vi "pulse_tester_16IQ.vi"() -> ()   [LabVIEW 2022 SP3]
uses:
  <vilib>/Analysis/NI_AALPro.lvlib
  <vilib>/measure/NI_MAPro.lvlib
  <vilib>/measure/maspectr.llb/FFT Power Spectrum and PSD for 1 Chan (CDB).vi
  <instrlib>/_niInstr/Basic Elements/v1/FPGA/niInstr Basic Elements v1 FPGA.lvlib
  emitter params.ctl
  pdw.ctl
  mode_type.ctl
panel:
  out "D phase to Dt":dbl[](graph)
  out "output valid":i16[](graph)
  in  "tx rate":i32=50
  out "Cluster":T1={"PW"=60000, "frequency shift"=0.004999999999999005, "amp"=0.31623077392578125, "mode type"=enum."LFM", "mode depth"=234562481, "mode filter"=0, "phase shift"=0.0}
  out "Array":i32[](array[numeric])
  out "free DDS":i16[](graph)
  out "Power Spectrum / PSD":cluster{"f0":dbl, "df":dbl, "magnitude":dbl[]}[](graph)
  out "amp out":dbl[](graph)
  out "phase out":dbl[](graph)
  in  "num of sampels for test":i32=65000 format="%.0p"
  out "I data":dbl[](graph)
  in  "emmiter":T3[](array[typedef])=[{"f set"=[1000000.0], "hop rate (Hz)"=6000.0, "d.c."=0.9, "amp (dB)"=-10.0, "mod type"=enum."LFM", "mod depth"=10000000.0, "DOA"=0.0, "t start"=0.0, "t end"=0.0}] {"t end" format="%#_3p"; "t start" format="%#_3p"; "DOA" format="%#_3p"; "mod depth" format="%.0p"}
  out "phase in to DDS":dbl[](graph)
  out "frequncy  in to DDS":dbl[](graph)
  in  "Fs":i32=200000000 format="%.0p"
  # "mode type:\n0- cw\n3-lfm\n4- bpsk\n5-qpsk"
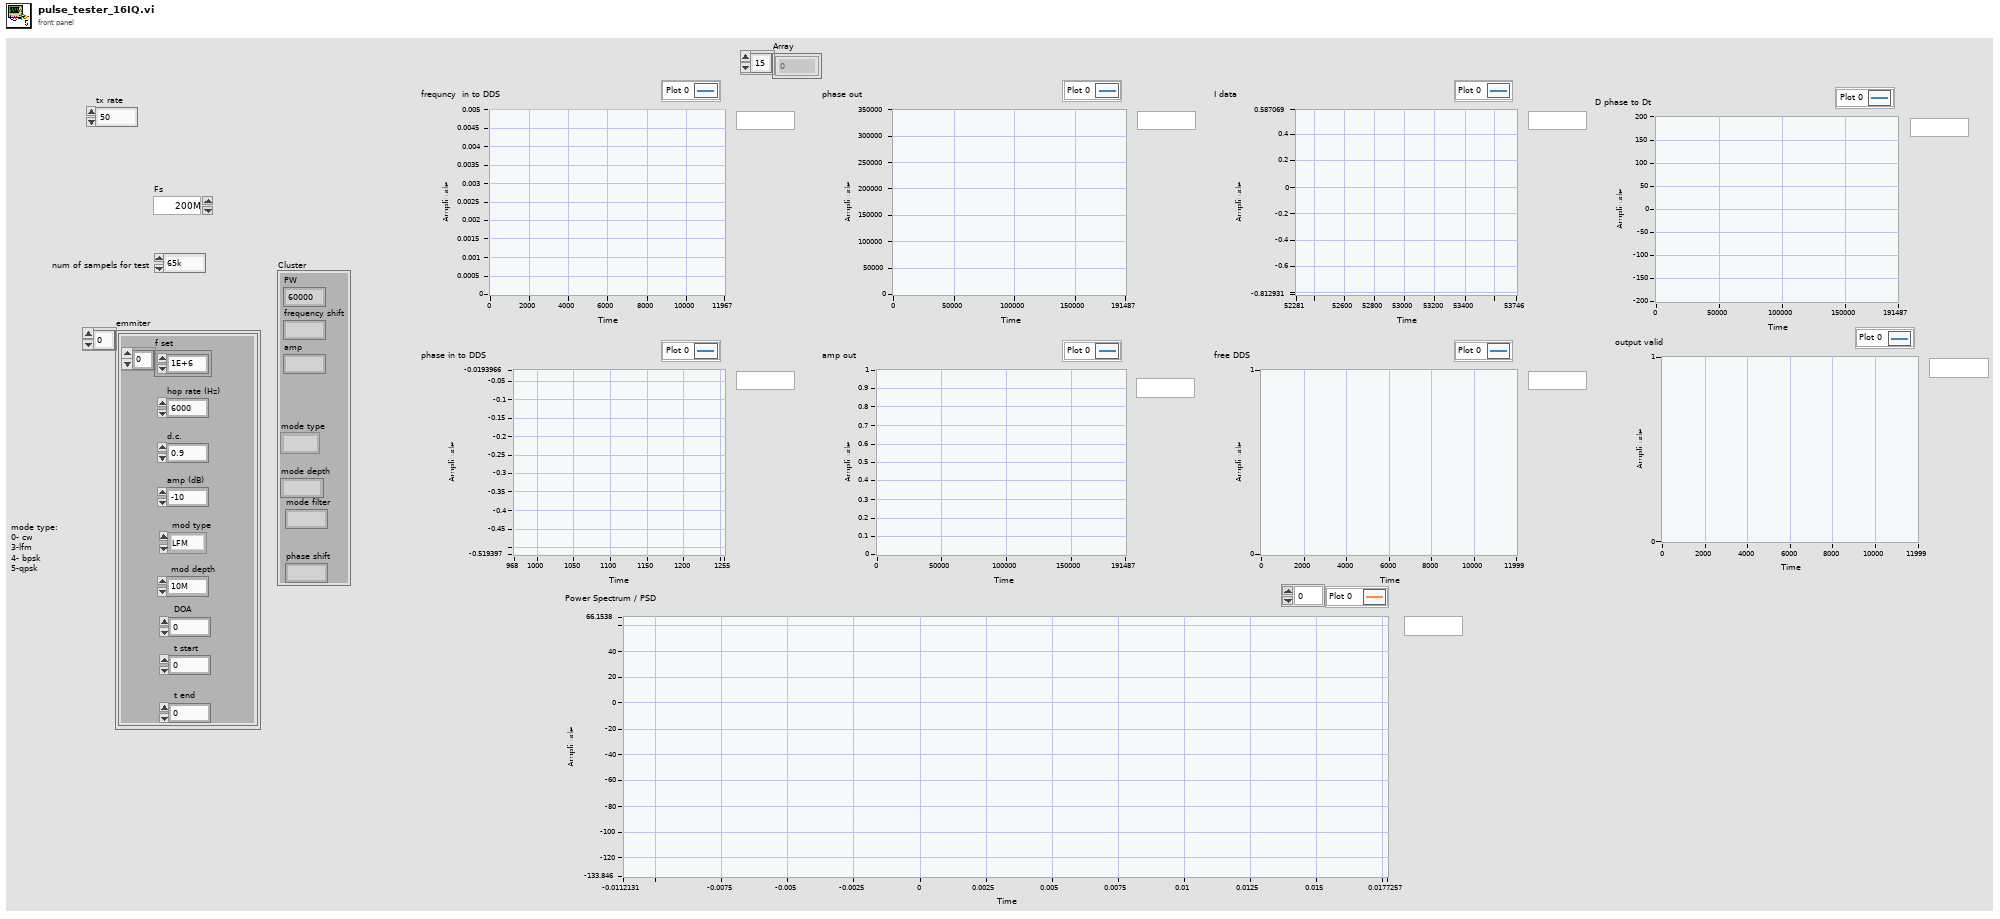
[diagram p1: front panel]
types:
  T1 = typedef "pdw.ctl" = cluster{"PW":u32, "frequency shift":fxp<+/-,48,0>, "amp":fxp<+/-,18,1>, "mode type":T2, "mode depth":u32, "mode filter":u8, "phase shift":fxp<+/-,16,1>}
  T2 = typedef "mode_type.ctl" = enum8{"CW", "NC - CW", "NC - cw", "LFM", "BPSK", "QPSK"}
  T3 = typedef "emitter params.ctl" = cluster{"f set":dbl[], "hop rate (Hz)":dbl, "d.c.":dbl, "amp (dB)":dbl, "mod type":T2, "mod depth":dbl, "DOA":dbl, "t start":dbl, "t end":dbl}
  T4 = typedef "PDW_lv2.ctl" = cluster{"t start":dbl, "frequency (Hz)":dbl, "duration (sec)":dbl, "amp (lin)":dbl, "mod type":T2, "mod depth":dbl, "phase":i32[]}
  T5 = typedef "niInstr DSP v1 Shared.lvlib/IQ Data.ctl" = cluster{"I":fxp<+/-,18,1>, "Q":fxp<+/-,18,1>, "overflow":bool}
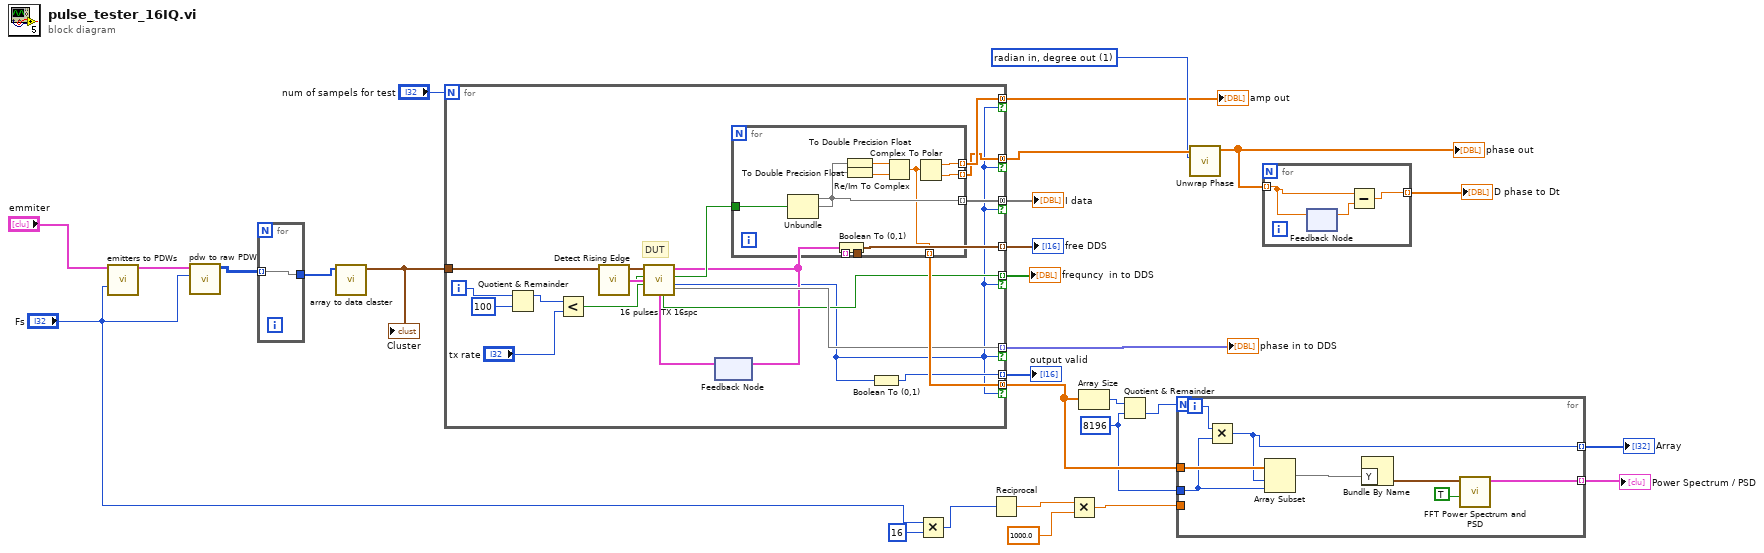
[diagram p0: block diagram]
diagram:
  w14 = 8196 ("length")
  w24 = 1 items=["radian in, radian out", "radian in, degree out", "degree in, degree out", "degree in, radian out"] ("phase unit")
  n1 = call "emitters to PDWs.vi"("emmiter"="emmiter", "center frequency (Hz)"="Fs") -> ("sorted array"=w21:T4[])  [unwired: 11 in, 2 out]
  n2 = call "pdw to raw PDW.vi"("Fs"="Fs", "PDWs"=w21) -> ("Array"=w8:u64[][])  [unwired: 7 in, 2 out]
  n3 = for {
    tunnel: [w29] -> w7
    tunnel: w8 -> [w29] mode=indexing
  }
  n4 = call "array to data claster.vi"("Array"=w7) -> ("Cluster"=w18:T1)  [unwired: 10 in]
  "Cluster" <- w18
  n5 = for {
    N: "num of sampels for test" -> [_]
    tunnel: [w47] -> w28 mode=concatenating if=w30
    tunnel: [w40] -> w27 mode=indexing if=w30
    tunnel: [w41] -> w26 mode=indexing if=w30
    tunnel: [w44] -> w25 mode=concatenating if=w30
    tunnel: [w45] -> w23 mode=concatenating if=w30
    tunnel: w18 -> [w46]
    tunnel: [w43] -> w20 mode=concatenating if=w30
    tunnel: [w42] -> w17 mode=indexing
    tunnel: [w33] -> w11 mode=indexing
    i -> [w38]
    # "DUT"
    n6 = Quotient & Remainder(x=w38, y=100) -> (x-y*floor(x/y)=w36:i32)  [unwired: 1 out]
    n7 = Less?(x=w36, y="tx rate") -> (x < y?=w34:bool)
    n8 = feedback #1() -> (w32:T5[])  [unwired: 1 in]
    n9 = call <instrlib>:"Detect Rising Edge.vi"("signal"=w32) -> ("edge detected"=w31:bool)  [unwired: 14 in]
    n10 = call "16 pulses TX 16spc.vi"("IQ_run"=w34, "PDW input Valid"=w31, "array PDW"=w46) -> ("fpga clock"=w30:u64, "output valid"=w48:bool, "IQ out"=w39:T5[], "ready for input"=w40:bool, 6:w41)  [unwired: 2 in, 2 out]
    n11 = feedback-in #1(w39) -> ()
    n12 = for {
      tunnel: w48 -> [w58]
      tunnel: [w57] -> w47 mode=indexing
      tunnel: [w55] -> w45 mode=indexing
      tunnel: [w54] -> w44 mode=indexing
      tunnel: [w53] -> w43 mode=indexing
      tunnel: [w52] -> w42
      tunnel: w39 -> [w49] mode=indexing
      n13 = Unbundle(w58) -> (w57, w56)  [unwired: 1 out]
      n14 = Boolean To (0,1)(Boolean=w49) -> (0, 1=w52:cluster{"I":i16, "Q":i16, "overflow":i16})
      n15 = To Double Precision Float(number=w57) -> (double precision float=w51:dbl)
      n16 = To Double Precision Float(number=w56) -> (double precision float=w50:dbl)
      n17 = Re/Im To Complex(1:w50, 2:w51) -> (0:w53:cdb)
      n18 = Complex To Polar(r * e^(i*theta)=w53) -> (r=w55:dbl, theta=w54:dbl)
    }
    n19 = Boolean To (0,1)(Boolean=w30) -> (0, 1=w33:i16)
  }
  "frequncy  in to DDS" <- w27
  "phase in to DDS" <- w26
  "I data" <- w28
  "amp out" <- w23
  "free DDS" <- w17
  "output valid" <- w11
  n20 = Multiply(x="Fs", y=16) -> (x*y=w4:i32)
  n21 = Reciprocal(x=w4) -> (1/x=w3:dbl)
  n22 = Multiply(x=w3, y=1000.0) -> (x*y=w1:dbl)
  n23 = Array Size(array=w20) -> (size(s)=w15:i32)
  n24 = Quotient & Remainder(x=w15, y=w14) -> (floor(x/y)=w13:i32)  [unwired: 1 out]
  n25 = for {
    N: w13 -> [_]
    tunnel: w20 -> [w63]
    tunnel: w1 -> [_]
    tunnel: w14 -> [w62]
    tunnel: [w60] -> w12 mode=indexing
    tunnel: [w61] -> w16 mode=indexing
    i -> [w59]
    n26 = Multiply(x=w59, y=w62) -> (x*y=w61:i32)
    n27 = Array Subset(array=w63, index=w61, length=w62) -> (w64:cdb[])
    n28 = Bundle By Name("Y"=w64) -> (w66:waveform(cdb))  [unwired: 1 in]
    n29 = call-poly <vilib>:"FFT Power Spectrum and PSD.vi"("dB On (F)"=TRUE, "time signal"=w66) -> ("Power Spectrum / PSD"=w60:cluster{"f0":dbl, "df":dbl, "magnitude":dbl[]})  [unwired: 6 in, 3 out]
  }
  "Power Spectrum / PSD" <- w12
  "Array" <- w16
  n30 = call <vilib>:"Unwrap Phase.vi"("phase unit"=w24, "Phase"=w25) -> ("Unwrapped Phase"=w10:dbl[])  [unwired: 8 in, 1 out]
  "phase out" <- w10
  n31 = for {
    tunnel: w10 -> [w69] mode=indexing
    tunnel: [w67] -> w9 mode=indexing
    n32 = feedback-in #2(w69) -> ()
    n33 = feedback #2() -> (w68:dbl)  [unwired: 1 in]
    n34 = Subtract(x=w69, y=w68) -> (x-y=w67:dbl)
  }
  "D phase to Dt" <- w9
